vi "Setup_Filepath.vi"(2 "Setup File Type":T1, 3 "Filename in":string) -> (0 "Filename Out":path, 1 "Directory":path)   [LabVIEW 2021]
uses:
  Setup_Filetype.ctl
  Globals/Constants_global.vi
  Globals/Preference_global.vi
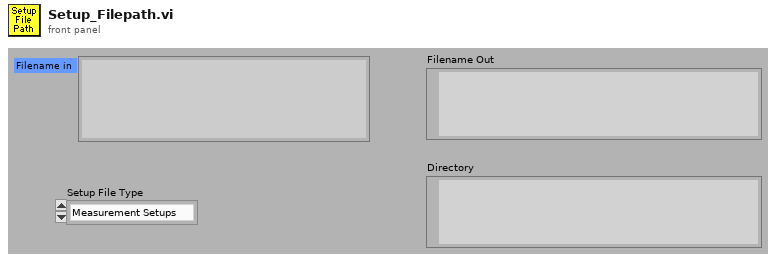
[diagram p1: front panel]
types:
  T1 = typedef "Setup_Filetype.ctl" = enum16{"Measurement Setups", "Calibration Setups", "General", "Results File Plotter Setups", "Speed Calib Tweaks"}
  T2 = typedef "LVDateTimeRec.ctl" = cluster{"fractional second":dbl, "second":i32, "minute":i32, "hour":i32, "day of month":i32, "month":i32, "year":i32, "day of week":i32, "day of year":i32, "DST":i32}
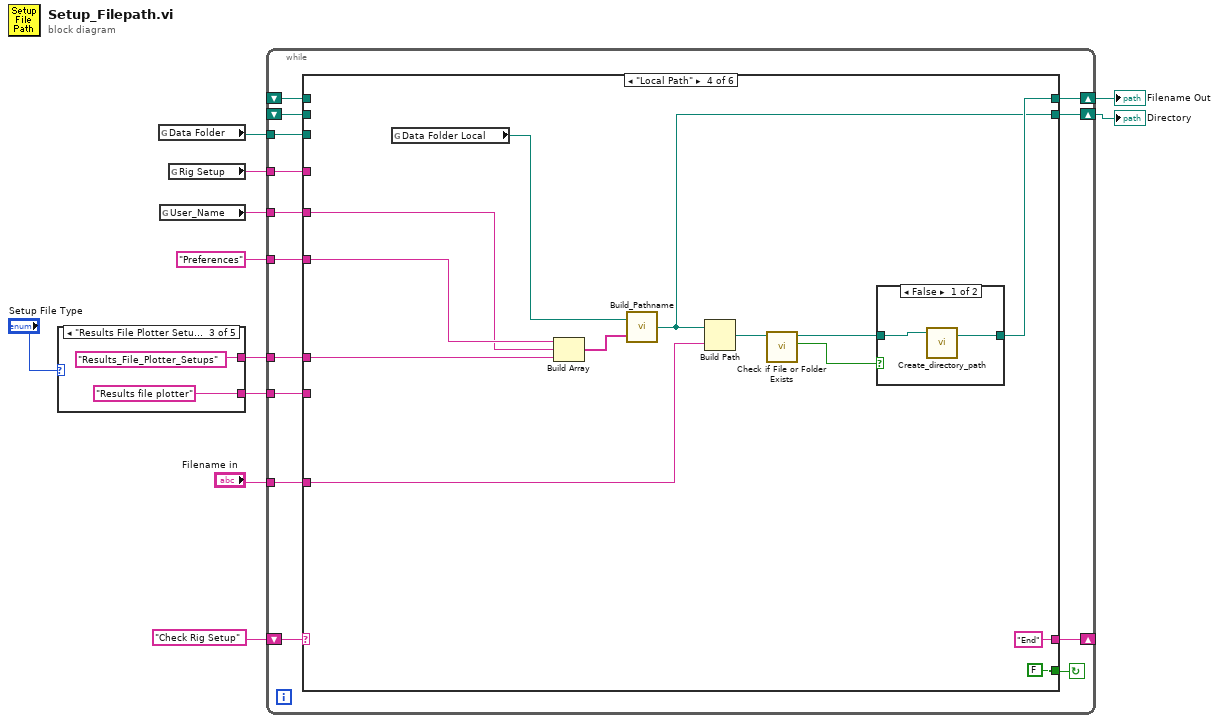
[diagram p0: block diagram]
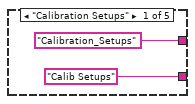
[diagram p2: hidden frame]
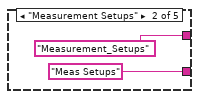
[diagram p3: hidden frame]
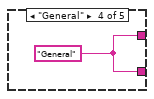
[diagram p4: hidden frame]
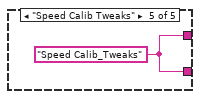
[diagram p5: hidden frame]
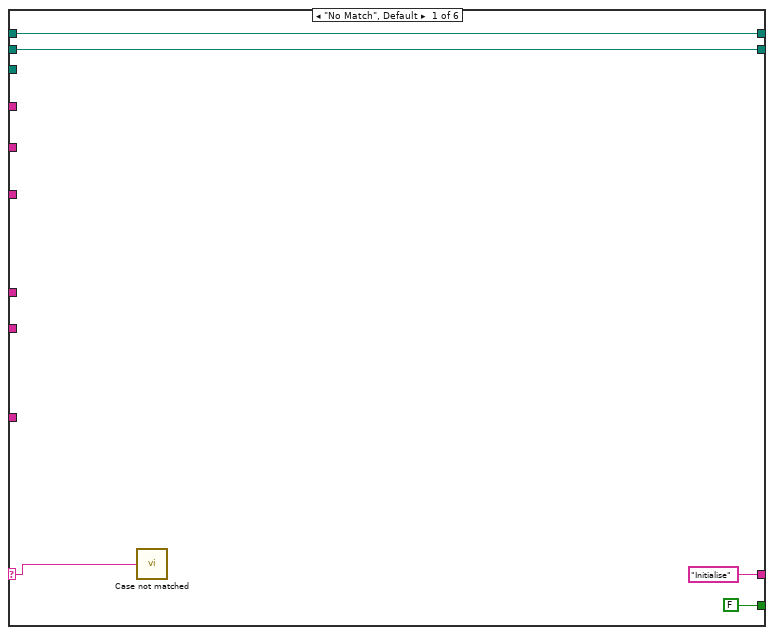
[diagram p6: hidden frame]
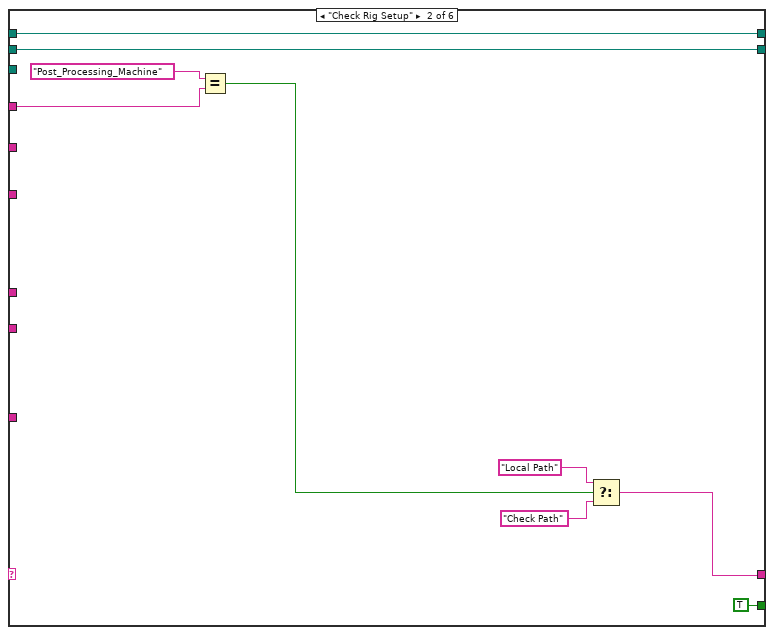
[diagram p7: hidden frame]
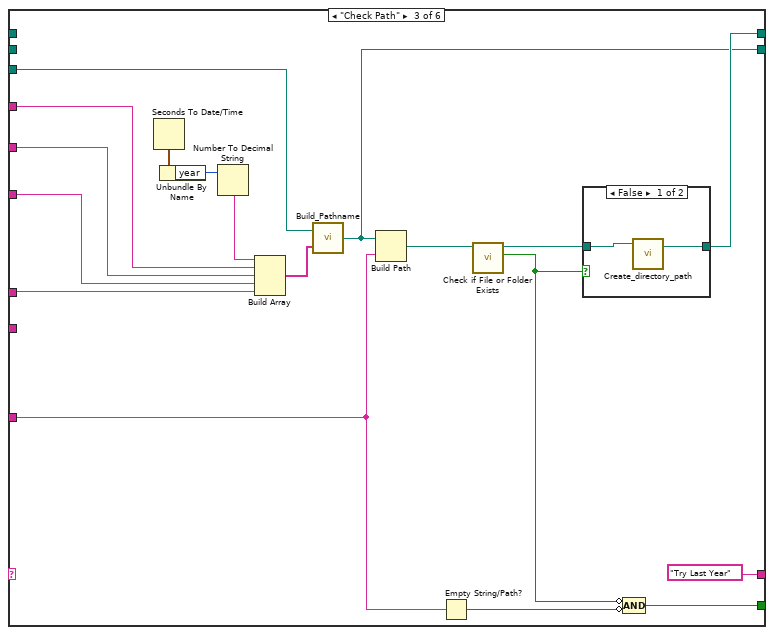
[diagram p8: hidden frame]
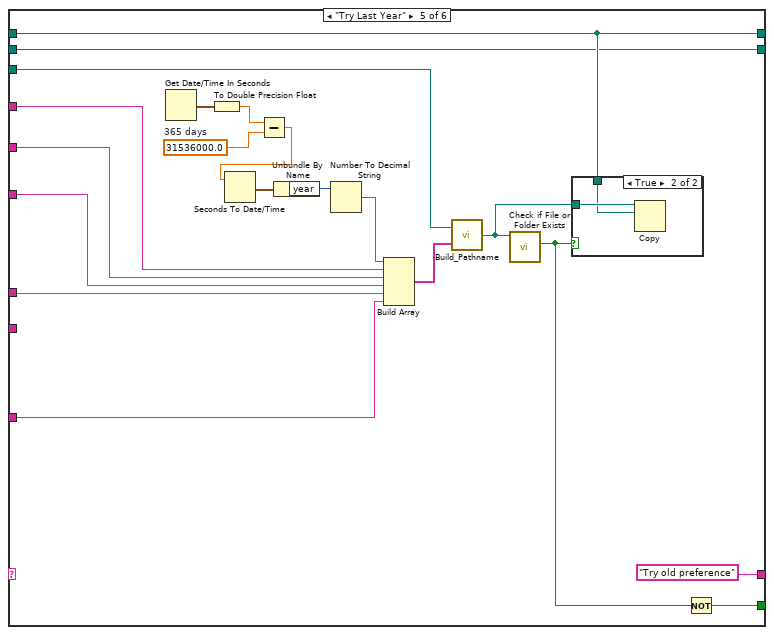
[diagram p11: hidden frame]
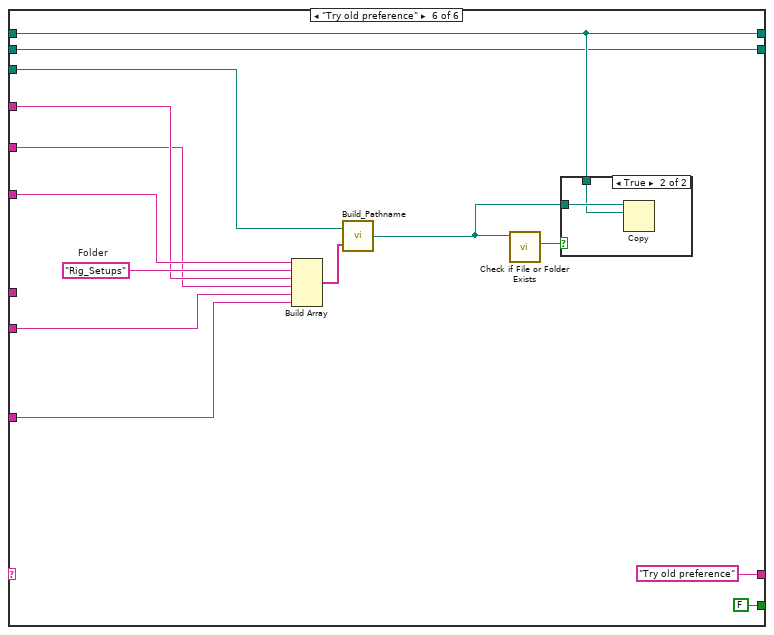
[diagram p13: hidden frame]
diagram:
  n1 = case shown="\"Results File Plotter Setups\"" "Setup File Type" {
    tunnel: ["Calibration_Setups" "Measurement_Setups" "Results_File_Plotter_Setups" w18 w19] -> w3
    tunnel: ["Calib Setups" ("name or relative path") "Meas Setups" ("name or relative path") "Results file plotter" ("name or relative path") w18 w19] -> w2
    frame "Calibration Setups" {
    }
    frame "Measurement Setups" {
    }
    frame "Results File Plotter Setups" {
    }
    frame "General" {
      w18 = "General" ("name or relative path")
    }
    frame "Speed Calib Tweaks" {
      w19 = "Speed Calib_Tweaks" ("name or relative path")
    }
  }
  n2 = global read "Constants_global.vi" "Data Folder"() -> (w10:path)
  n3 = global read "Preference_global.vi" "User_Name"() -> (w8:string)
  n4 = global read "Preference_global.vi" "Rig Setup"() -> (w9:string)
  n5 = while {
    shift-left: "Check Rig Setup" -> [w31]
    shift-right: [w32] -> _
    tunnel: w3 -> [w30]
    tunnel: w10 -> [w29]
    tunnel: w9 -> [w28]
    tunnel: w8 -> [w27]
    tunnel: "Filename in" -> [w26]
    shift-right: [w25] -> w6
    shift-left: _ -> [w24]
    tunnel: "Preferences" ("name or relative path") -> [w23]
    tunnel: w2 -> [w22]
    shift-right: [w21] -> w1
    shift-left: _ -> [w20]
    stop <- w33 continue-if-true
    n6 = case shown="\"Local Path\"" w31 {
      selector: w31 -> [w34 _ _ _ _ _]
      tunnel: [FALSE TRUE w53 FALSE w97 FALSE] -> w33
      tunnel: ["Initialise" w40 "Try Last Year" "End" "Try old preference" "Try old preference"] -> w32
      tunnel: w30 -> [_ _ w63 w71 w102 _]
      tunnel: w29 -> [_ _ w62 _ w101 w118]
      tunnel: w28 -> [_ w46 w61 _ w100 w114]
      tunnel: w27 -> [_ _ w60 w72 w99 w113]
      tunnel: w26 -> [_ _ w56 w77 w98 w109]
      tunnel: [w36 w43 w58 w79 w91 w112] -> w25
      tunnel: w24 -> [w36 w43 _ _ w91 w112]
      tunnel: w23 -> [_ _ w52 w73 w90 w116]
      tunnel: w22 -> [_ _ _ _ _ w108]
      tunnel: [w35 w39 w48 w75 w85 w107] -> w21
      tunnel: w20 -> [w35 w39 _ _ w85 w107]
      frame "No Match", Default {
        n7 = call "Case not matched.vi"("Case Name not Matched"=w34) -> ()
      }
      frame "Check Rig Setup" {
        n8 = Equal?(x="Post_Processing_Machine" ("Rig Setup"), y=w46) -> (x = y?=w45:bool)
        n9 = Select(t="Local Path", s=w45, f="Check Path") -> (s? t:f=w40:string)
      }
      frame "Check Path" {
        n10 = Seconds To Date/Time() -> (date time rec=w51:T2)  [unwired: 2 out]
        n11 = Unbundle By Name(w51) -> ("year"=w50:i32)
        n12 = Number To Decimal String(number=w50) -> (decimal integer string=w49:string)  [unwired: 1 out]
        n13 = Build Array(w49, w61, w60, w52, w63) -> (w64:string[])
        n14 = call "Build_Pathname.vi"("PathElements"=w64, "PathnameIn"=w62) -> ("AppendedPath"=w48:path)
        n15 = Build Path(base path=w48, name or relative path=w56) -> (appended path=w57:path)
        n16 = Empty String/Path?(string/path=w56) -> (empty?=w54:bool)
        n17 = call <vilib>:"Check if File or Folder Exists.vi"("path"=w57) -> ("file or folder exists?"=w55:bool, "dup path"=w59:path)  [unwired: 1 in, 8 out]
        n18 = case shown="False" w55 {
          tunnel: w59 -> [w67 w68]
          tunnel: [w66 w68] -> w58
          frame False {
            n19 = call "Create_directory_path.vi"("Path name"=w67) -> ("Path name Out"=w66:path)  [unwired: 2 in, 1 out]
          }
          frame True {
          }
        }
        n20 = Compound Arithmetic op=AND(invert w55, invert w54) -> (w53:bool)
      }
      frame "Local Path" {
        n21 = global read "Constants_global.vi" "Data Folder Local"() -> (w74:path)
        n22 = Build Array(w73, w72, w71) -> (w81:string[])
        n23 = call "Build_Pathname.vi"("PathElements"=w81, "PathnameIn"=w74) -> ("AppendedPath"=w75:path)
        n24 = Build Path(base path=w75, name or relative path=w77) -> (appended path=w78:path)
        n25 = call <vilib>:"Check if File or Folder Exists.vi"("path"=w78) -> ("file or folder exists?"=w76:bool, "dup path"=w80:path)  [unwired: 1 in, 8 out]
        n26 = case shown="False" w76 {
          tunnel: w80 -> [w83 w84]
          tunnel: [w82 w84] -> w79
          frame False {
            n27 = call "Create_directory_path.vi"("Path name"=w83) -> ("Path name Out"=w82:path)  [unwired: 2 in, 1 out]
          }
          frame True {
          }
        }
      }
      frame "Try Last Year" {
        w94 = 31536000.0  # 365 days
        n28 = Get Date/Time In Seconds() -> (seconds since 1Jan1904=w95:timestamp)
        n29 = To Double Precision Float(number=w95) -> (double precision float=w96:dbl)
        n30 = Subtract(x=w96, y=w94) -> (x-y=w87:dbl)
        n31 = Seconds To Date/Time(time stamp (now)=w87) -> (date time rec=w89:T2)  [unwired: 1 out]
        n32 = Unbundle By Name(w89) -> ("year"=w88:i32)
        n33 = Number To Decimal String(number=w88) -> (decimal integer string=w86:string)  [unwired: 1 out]
        n34 = Build Array(w86, w100, w99, w90, w102, w98) -> (w103:string[])
        n35 = call "Build_Pathname.vi"("PathElements"=w103, "PathnameIn"=w101) -> ("AppendedPath"=w93:path)
        n36 = call <vilib>:"Check if File or Folder Exists.vi"("path"=w93) -> ("file or folder exists?"=w92:bool)  [unwired: 1 in, 9 out]
        n37 = case shown="True" w92 {
          tunnel: w93 -> [_ w106]
          tunnel: w91 -> [_ w105]
          frame False {
          }
          frame True {
            n38 = Copy(10:w105, 11:w106) -> ()  [unwired: 3 in, 3 out]
          }
        }
        n39 = Not(x=w92) -> (.not. x?=w97:bool)
      }
      frame "Try old preference" {
        w115 = "Rig_Setups"  # Folder
        n40 = Build Array(w116, w115, w114, w113, w108, w109) -> (w119:string[])
        n41 = call "Build_Pathname.vi"("PathElements"=w119, "PathnameIn"=w118) -> ("AppendedPath"=w110:path)
        n42 = call <vilib>:"Check if File or Folder Exists.vi"("path"=w110) -> ("file or folder exists?"=w117:bool)  [unwired: 1 in, 9 out]
        n43 = case shown="True" w117 {
          tunnel: w110 -> [_ w122]
          tunnel: w112 -> [_ w121]
          frame False {
          }
          frame True {
            n44 = Copy(10:w121, 11:w122) -> ()  [unwired: 3 in, 3 out]
          }
        }
      }
    }
  }
  "Filename Out" <- w6
  "Directory" <- w1
